vi "motor_driver_data_acquisition.vi"() -> ()   [LabVIEW 2014]
uses:
  <vilib>/DAQmx/write.llb/DAQmx Write (Digital 1D Bool 1Chan 1Samp).vi
  <vilib>/DAQmx/create/channels.llb/DAQmx Create Channel (DO-Digital Output).vi
  <vilib>/DAQmx/miscellaneous.llb/DAQmx Fill In Error Info.vi
panel:
  out "Mean (DC)":dbl
  in  "Boolean":bool caption="left- anticlockwise \nright- clockwise"
  out "Angle":dbl
  out "Mean DC -angle":cluster{"Y":dbl[], "Y":dbl[]}[](graph)
  out "Waveform Graph":dynamicdata(graph)
  in  "stop":bool
  in  "Lines":tag="Dev1/port0/line0:7"
  in  "Array":fxp<+,64,4>[][](array[numeric])
  out "Boolean array 2":bool[](array[boolean])
  out "Iterations":i32
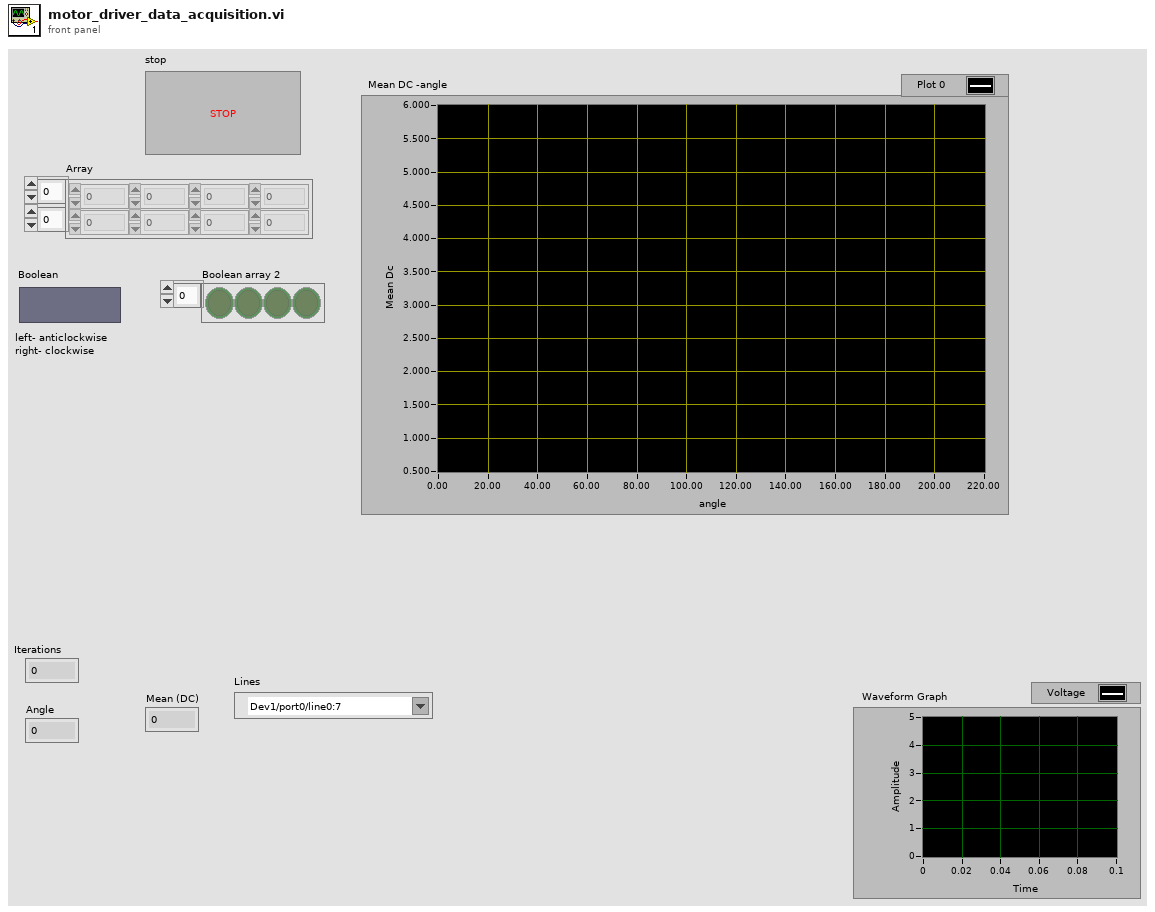
[diagram p1: front panel]
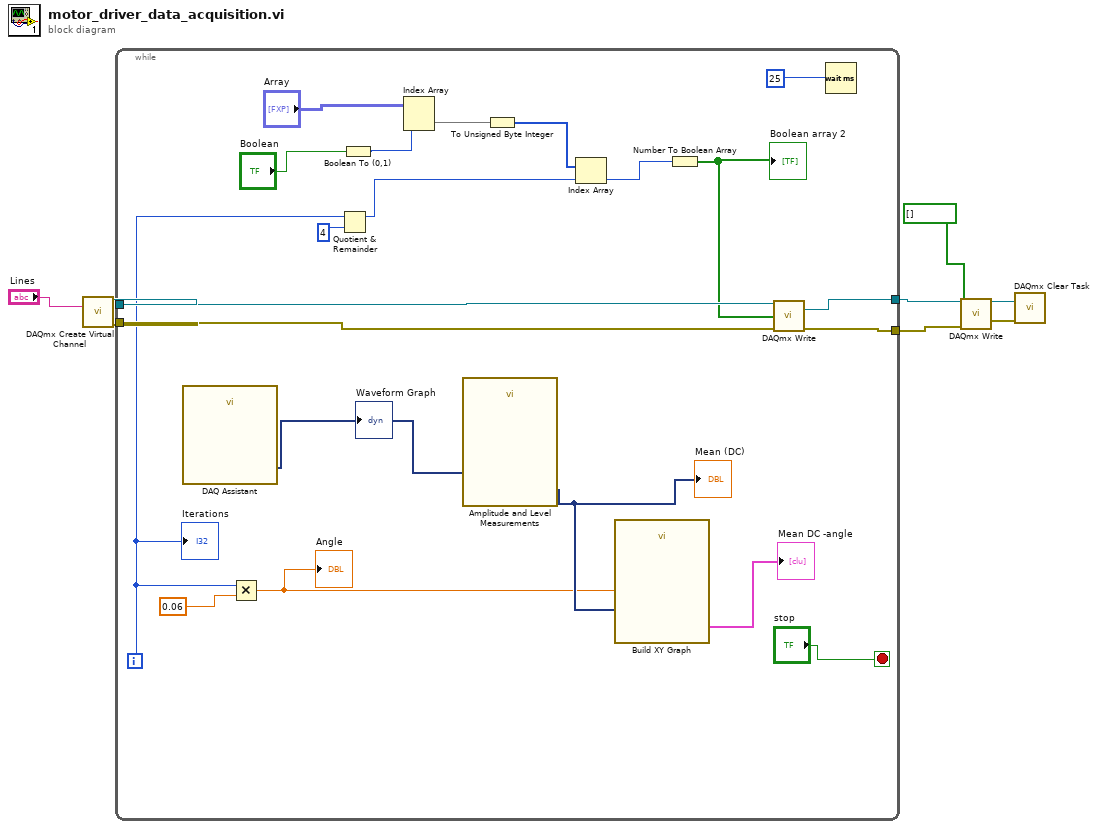
[diagram p0: block diagram]
diagram:
  n1 = call-poly <vilib>:"DAQmx Create Virtual Channel.vi"("lines"="Lines") -> ("task out"=w8:refnum<k21>, "error out"=w7:errorcluster)  [unwired: 13 in]
  n2 = while {
    tunnel: [w26] -> w5
    tunnel: w8 -> [w25]
    tunnel: w7 -> [w24]
    tunnel: [w23] -> w2
    i -> [w16]
    stop <- "stop" stop-if-true
    n3 = call "DAQ Assistant"() -> ("data"=w17:dynamicdata)  [unwired: 16 in, 3 out]
    "Waveform Graph" <- w17
    n4 = Multiply(x=w16, y=0.06) -> (x*y=w9:dbl)
    "Angle" <- w9
    n5 = Quotient & Remainder(x=w16, y=4) -> (x-y*floor(x/y)=w28:i32)  [unwired: 1 out]
    n6 = Boolean To (0,1)(Boolean="Boolean") -> (0, 1=w12:i16)
    n7 = Index Array(array="Array", index (row)=w12) -> (element=w13:fxp<+,64,4>[])  [unwired: 1 in]
    n8 = call "Amplitude and Level Measurements"("Signals"=w17) -> ("Mean (DC)"=w10:dynamicdata)  [unwired: 13 in, 1 out]
    "Mean (DC)" <- w10
    n9 = To Unsigned Byte Integer(number=w13) -> (unsigned 8bit integer=w22:u8[])
    n10 = Index Array(array=w22, index=w28) -> (element=w27:u8)
    n11 = call "Build XY Graph"("Y Input"=w10, "X Input"=w9) -> ("XY Graph"=→"Mean DC -angle":cluster{"X":dbl[], "Y":dbl[]}[])  [unwired: 8 in, 1 out]
    n12 = Number To Boolean Array(number=w27) -> (Boolean array=w21:bool[])
    "Boolean array 2" <- w21
    n13 = call-poly <vilib>:"DAQmx Write.vi"("task/channels in"=w25, "data"=w21, "error in"=w24) -> ("task out"=w26:refnum<k21>, "error out"=w23:errorcluster)  [unwired: 10 in, 1 out]
    n14 = Wait (ms)(milliseconds to wait=u32 25 ("millisecond timer value")) -> ()  [unwired: 1 out]
    "Iterations" <- w16
  }
  n15 = call-poly <vilib>:"DAQmx Write.vi"("task/channels in"=w5, "data"=bool[] [], "error in"=w2) -> ("task out"=w4:refnum<k21>, "error out"=w3:errorcluster)  [unwired: 10 in, 1 out]
  n16 = call <vilib>:"DAQmx Clear Task.vi"("task in"=w4, "error in"=w3) -> ()  [unwired: 13 in, 1 out]
